vi "OpenVIs.vi"(8 "error in (no error)":errorcluster, 9 "Title Prefix In":string, 10 "VI Screenshots":T1, 11 "VI Path":path) -> (0 "error out":errorcluster, 2 "VI Screenshots out":T1, 5 "VI exists?":bool=TRUE)   [LabVIEW 2017]
uses:
  FilePaths.ctl
  Screenshots/Screenshot Type.ctl
  Screenshots/ScreenshotInfo.ctl
  Screenshots/VIScreenshots.ctl
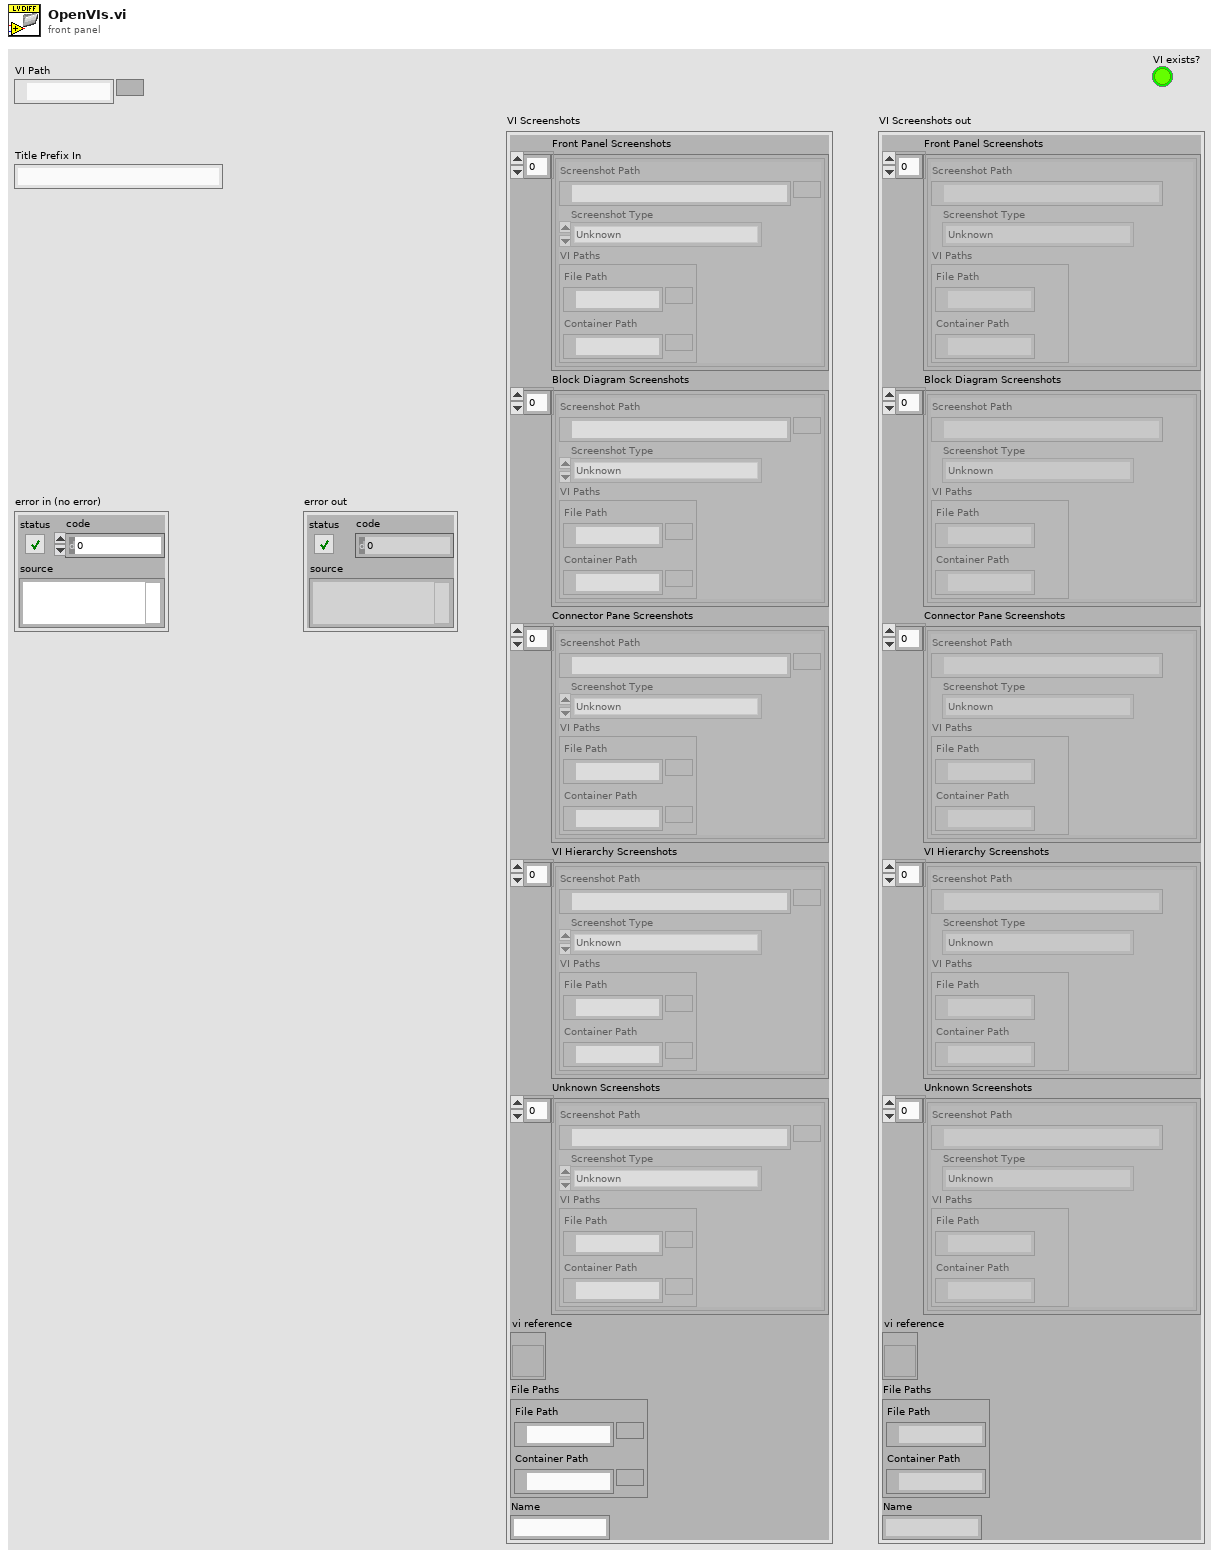
[diagram p1: front panel]
types:
  T1 = typedef "VIScreenshots.ctl" = cluster{"Front Panel Screenshots":T2[], "Block Diagram Screenshots":T2[], "Connector Pane Screenshots":T2[], "VI Hierarchy Screenshots":T2[], "Unknown Screenshots":T2[], "vi reference":refnum<vi>, "File Paths":cluster{"File Path":path, "Container Path":path}, "Name":string}
  T2 = typedef "ScreenshotInfo.ctl" = cluster{"Screenshot Path":path, "Screenshot Type":T3, "VI Paths":T4}
  T3 = typedef "Screenshot Type.ctl" = enum16{"Unknown", "Front Panel", "Connector Pane", "Block Diagram", "VI Hierarchy"}
  T4 = typedef "FilePaths.ctl" = cluster{"File Path":path, "Container Path":path}
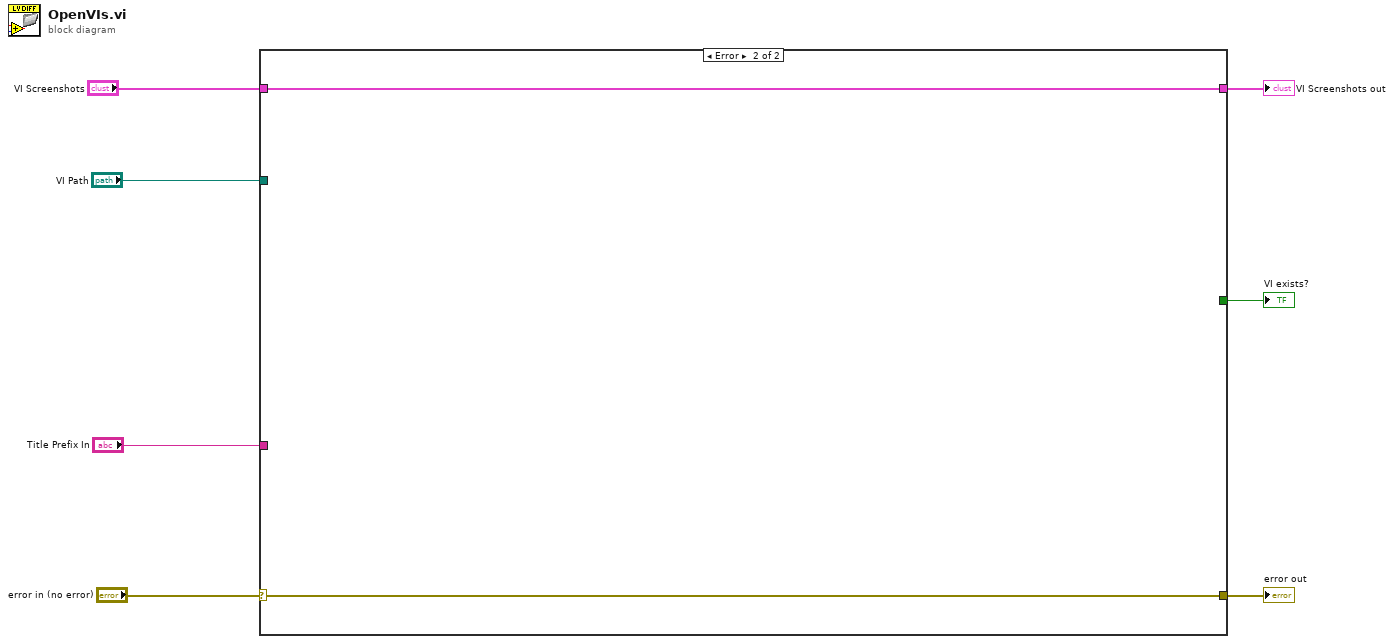
[diagram p0: block diagram]
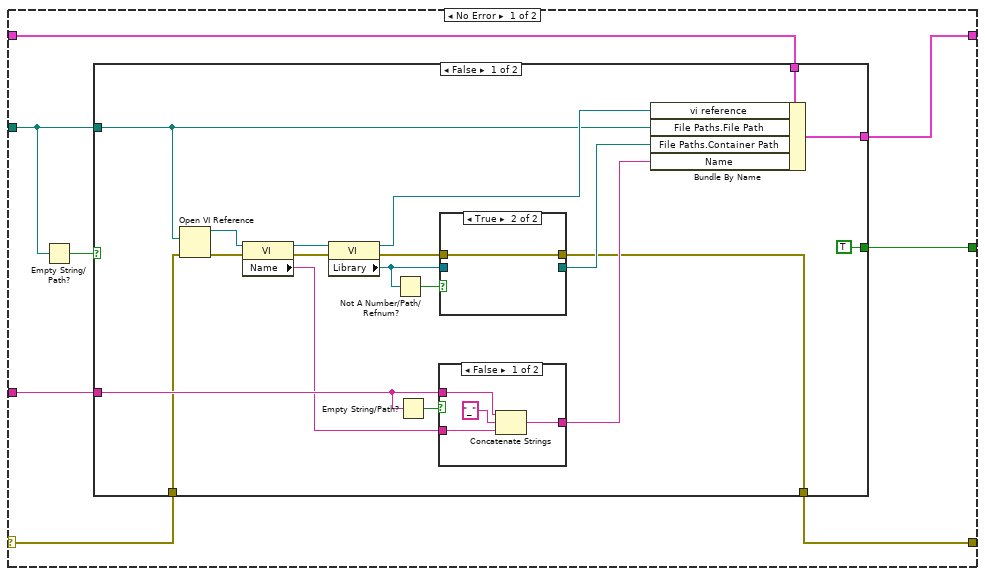
[diagram p2: hidden frame]
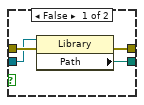
[diagram p4: hidden frame]
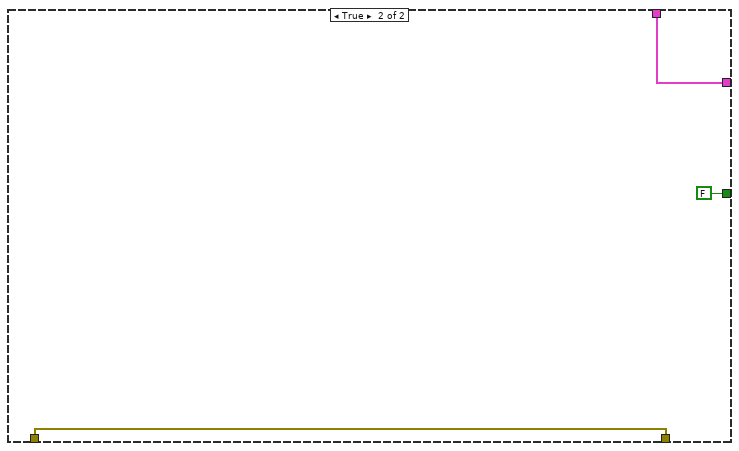
[diagram p5: hidden frame]
diagram:
  n1 = case shown="Error" "error in (no error)" {
    selector: "error in (no error)" -> [w9 w49]
    tunnel: [w12 w49] -> w6
    tunnel: "VI Screenshots" -> [w15 w48]
    tunnel: [w14 w48] -> w4
    tunnel: "VI Path" -> [w11 _]
    tunnel: "Title Prefix In" -> [w13 _]
    tunnel: [w8 _] -> w1
    frame No Error {
      n2 = Empty String/Path?(string/path=w11) -> (empty?=w10:bool)
      n3 = case shown="False" w10 {
        tunnel: w15 -> [w31 w47]
        tunnel: [w29 w47] -> w14
        tunnel: w13 -> [w22 _]
        tunnel: [w19 w46] -> w12
        tunnel: w11 -> [w18 _]
        tunnel: w9 -> [w17 w46]
        tunnel: [TRUE FALSE] -> w8
        frame False {
          n4 = Open VI Reference(vi path=w18, error in (no error)=w17) -> (vi reference=w28:refnum<vi>, error out=w27:errorcluster)  [unwired: 4 in]
          n5 = property class="VI"(reference=w28, error in=w27) -> (reference out=w25:refnum<vi>, error out=w26:errorcluster, "Name"=w21:string)
          n6 = property class="VI"(reference=w25, error in=w26) -> (reference out=w24:refnum<vi>, error out=w34:errorcluster, "Library"=w32:refnum<vi>)
          n7 = Not A Number/Path/Refnum?(number/path/refnum=w32) -> (NaN/Path/Refnum?=w33:bool)
          n8 = Empty String/Path?(string/path=w22) -> (empty?=w23:bool)
          n9 = case shown="False" w23 {
            tunnel: w21 -> [w38 w39]
            tunnel: [w37 w39] -> w20
            tunnel: w22 -> [w35 _]
            frame False {
              n10 = Concatenate Strings(w35, "_" ("string"), w38) -> (w37:string)
            }
            frame True {
            }
          }
          n11 = case shown="True" w33 {
            tunnel: [w43 _] -> w30
            tunnel: w34 -> [w42 w44]
            tunnel: [w41 w44] -> w19
            tunnel: w32 -> [w40 _]
            frame False {
              n12 = property class="Library"(reference=w40, error in=w42) -> (error out=w41:errorcluster, "Path"=w43:path)  [unwired: 1 out]
            }
            frame True {
            }
          }
          n13 = Bundle By Name(cluster=w31, "vi reference"=w24, "File Paths.File Path"=w18, "File Paths.Container Path"=w30, "Name"=w20) -> (w29:T1)
        }
        frame True {
        }
      }
    }
    frame Error {
    }
  }
  "error out" <- w6
  "VI Screenshots out" <- w4
  "VI exists?" <- w1
